vi "Pipe Colors.vi"(11 "True Color":u32(colorbox)) -> (3 "Colors[4]":cluster{"FG":u32, "BG":u32}[](array[cluster]))   [LabVIEW 2022 SP3, in "Pipes.lvlib"]
uses:
  Pipes.lvlib
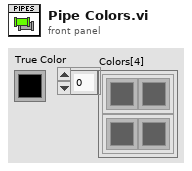
[diagram p1: front panel]
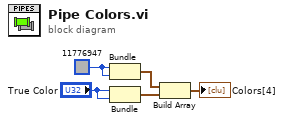
[diagram p0: block diagram]
diagram:
  w4 = u32 11776947
  n1 = Bundle(w4, w4) -> (w3:cluster{u32, u32})  [unwired: 1 in]
  n2 = Bundle("True Color"="True Color", "True Color"="True Color") -> (w5:cluster{"True Color":u32, "True Color":u32})  [unwired: 1 in]
  n3 = Build Array(w3, w5) -> (→"Colors[4]":cluster{"True Color":u32, "True Color":u32}[])
